vi "Initialize_Msg_Queue_FGV.vi"(8 "error in (no error)":errorcluster) -> (0 "error out":errorcluster)   [LabVIEW 2024, in "MANUAL_MODE.lvlib"]
doc: "ThisVI\n---------------------------------\nInitialize_Queue_FGV\n---------------------------------\n-initialize the FGV Message Queue"
uses:
  MANUAL_MODE.lvlib
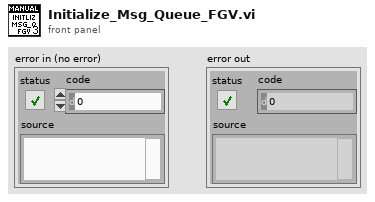
[diagram p1: front panel]
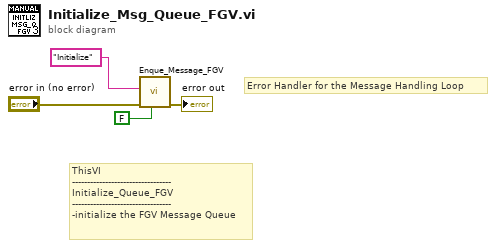
[diagram p0: block diagram]
diagram:
  # "Error Handler for the Message Handling Loop"
  # "ThisVI\n---------------------------------\nInitialize_Queue_FGV\n---------------------------------\n-initialize the FGV Message Queue"
  n1 = call "Enque_Message_FGV.vi"("Priority"=FALSE, "error in (no error)"="error in (no error)", "Message"="Initialize") -> ("error out"=→"error out":errorcluster)  [unwired: 8 in]
